vi "Display Thermocouple Data.vi"(0 "Sensor":T1={"Sensor Name"="AI 0", "Sensor Info"={"Manufacturer"="", "Model"="", "Serial Number"=""}, "Last Cal Info"={"Last Calibration Date"=3153138208.25, "Calibrator"="", "Cal Duration"=0}, "Voltage Range"={"High Limit"=0.0, "Low Limit"=10.0}, "EGU Range"={"High Limit"=0.0, "Low Limit"=10.0}, "Units"="Volts", "Calibration Type"=enum."Calibrate Analog", "EGU List"=[0.0, 10000.0], "Voltage List"=[0.0, 5.0], "Coefficients"=[3.658184866139891e-14, 1999.9999999999998], "Order"=1, "Algorithm"=enum."SVD", "Max Error % of Full Scale"=0.0, "Max Mean Squared Error"=0.0, "Use Error %"=FALSE, "Use MSE"=FALSE, "Allow Manual Entry"=FALSE, "Max Stability Error"=2.0, "Max Error % of Reading"=0.0, "Use Error % of Reading"=FALSE}, 1 "Shunt Cal":bool=TRUE, 5 "Channel Info":T2, 9 "Channel":string) -> (4 "Sensor out":T1)   [LabVIEW 2019]
uses:
  AI Read (waveform).vi
  AI Read (scaled array).vi
  <vilib>/Analysis/NI_AALBase.lvlib
  <vilib>/Analysis/baseanly.llb/Mean (DBL).vi
  <vilib>/Analysis/NI_AALPro.lvlib
  Type Defs and Controls/Channel Config Screen.ctl
panel:
  in  "Auto Shunt Cal Message":bool
  out "Temperature":dbl
  in  "OK":bool
  out "Sensor":string
  out "Channel Name":string
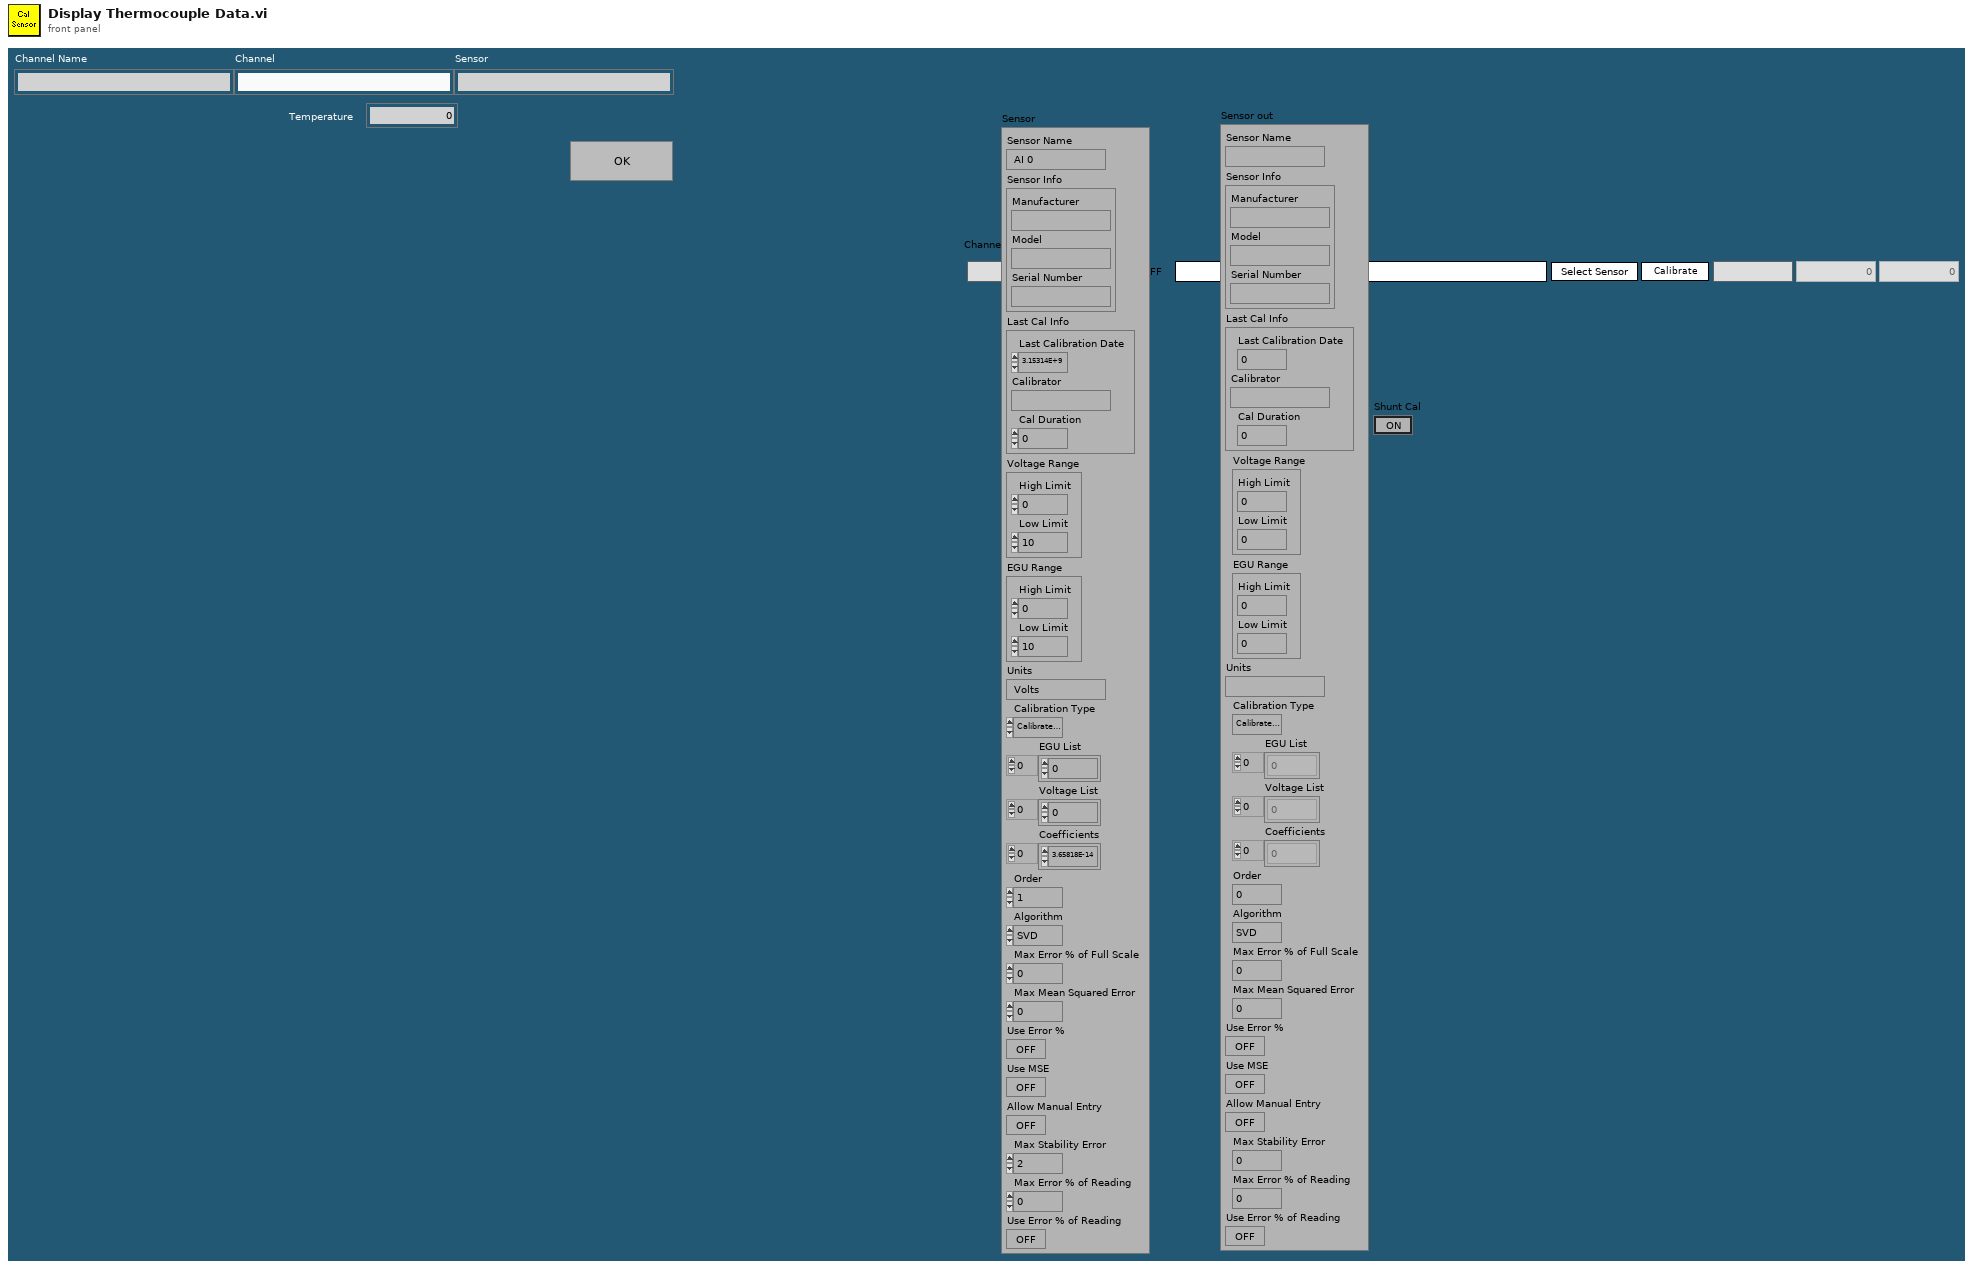
[diagram p1: front panel]
types:
  T1 = cluster{"Sensor Name":string, "Sensor Info":cluster{"Manufacturer":string, "Model":string, "Serial Number":string}, "Last Cal Info":cluster{"Last Calibration Date":dbl, "Calibrator":string, "Cal Duration":i32}, "Voltage Range":cluster{"High Limit":dbl, "Low Limit":dbl}, "EGU Range":cluster{"High Limit":dbl, "Low Limit":dbl}, "Units":string, "Calibration Type":enum16{"Calibrate Analog", "Compare Analog Calibration"}, "EGU List":dbl[], "Voltage List":dbl[], "Coefficients":dbl[], "Order":i32, "Algorithm":enum32{"SVD", "Givens", "Givens2", "Householder", "LU Decomposition", "Cholesky"}, "Max Error % of Full Scale":dbl, "Max Mean Squared Error":dbl, "Use Error %":bool, "Use MSE":bool, "Allow Manual Entry":bool, "Max Stability Error":dbl, "Max Error % of Reading":dbl, "Use Error % of Reading":bool}
  T2 = typedef "Channel Config Screen.ctl" = cluster{"Channel":string, "Description":string, "Acquire":bool, "Sensor":string, "Chg Sensor":bool, "Cal Date":string, "Offset":dbl, "Span":dbl, "Cal":bool, "Test Limits":bool, "Type":string, "Data Index":u32}
  T3 = cluster{"Channel Info":T2, "Channel":string, "Sensor":cluster{"Sensor Name":string, "Sensor Info":cluster{"Manufacturer":string, "Model":string, "Serial Number":string}, "Last Cal Info":cluster{"Last Calibration Date":dbl, "Calibrator":string, "Cal Duration":i32}, "Voltage Range":cluster{"High Limit":dbl, "Low Limit":dbl}, "EGU Range":cluster{"High Limit":dbl, "Low Limit":dbl}, "Units":string, "Calibration Type":enum16{"Calibrate Analog", "Compare Analog Calibration"}, "EGU List":dbl[], "Voltage List":dbl[], "Coefficients":dbl[], "Order":i32, "Algorithm":enum32{"SVD", "Givens", "Givens2", "Householder", "LU Decomposition", "Cholesky"}, "Max Error % of Full Scale":dbl, "Max Mean Squared Error":dbl, "Use Error %":bool, "Use MSE":bool, "Allow Manual Entry":bool, "Max Stability Error":dbl, "Max Error % of Reading":dbl, "Use Error % of Reading":bool}, "taskID":u32, "Allow Shunt Cal":bool}
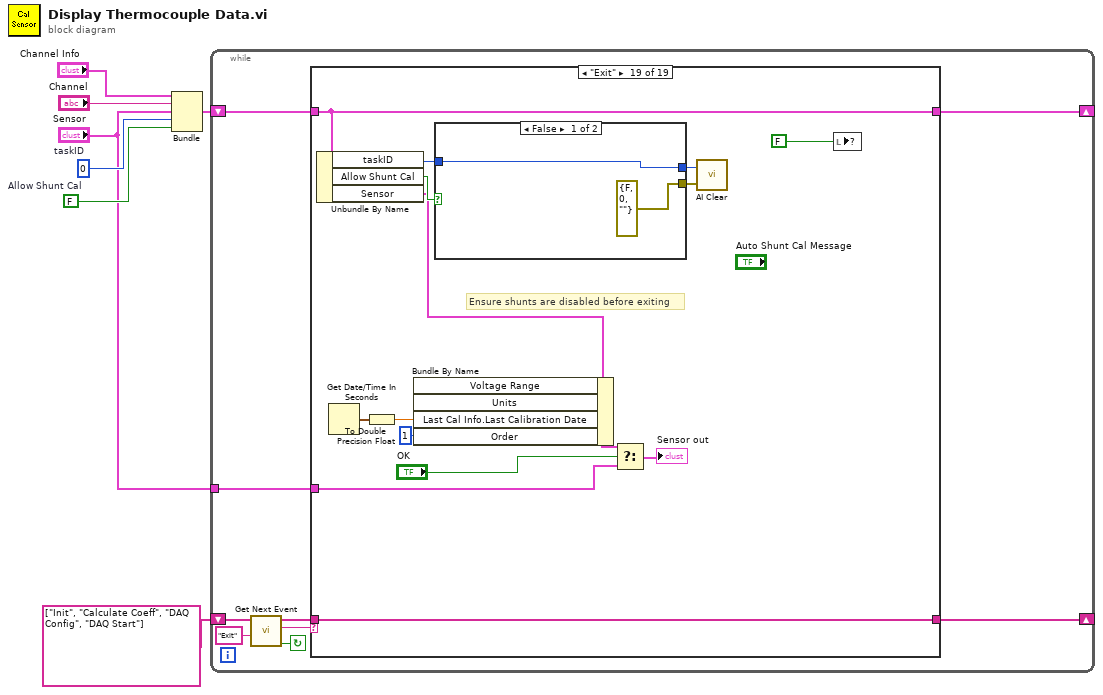
[diagram p0: block diagram]
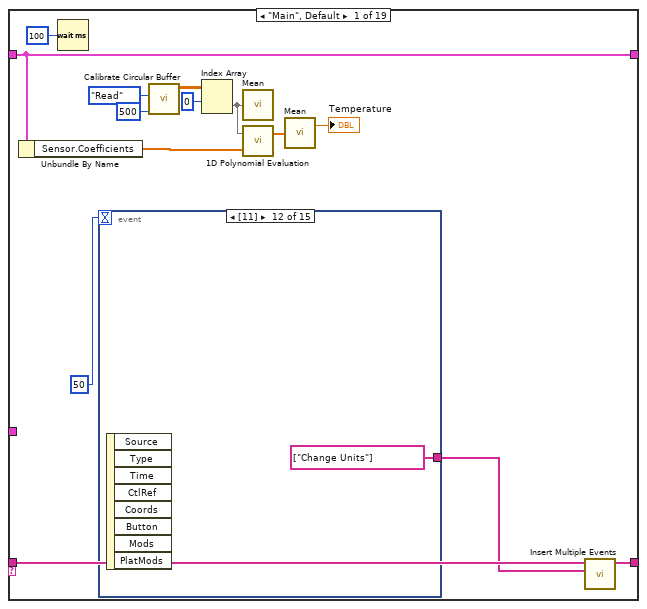
[diagram p2: hidden frame]
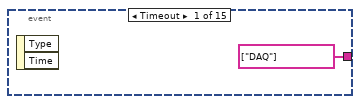
[diagram p3: hidden frame]
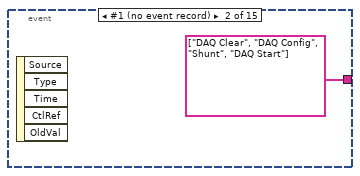
[diagram p4: hidden frame]
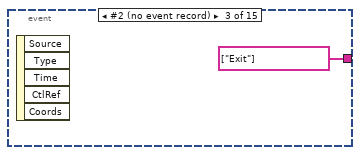
[diagram p5: hidden frame]
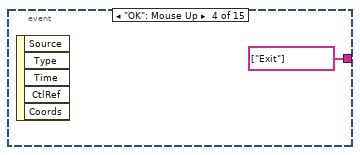
[diagram p6: hidden frame]
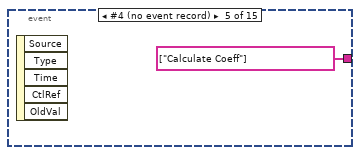
[diagram p7: hidden frame]
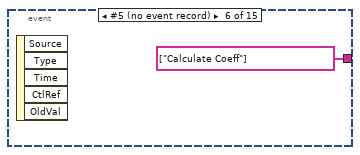
[diagram p8: hidden frame]
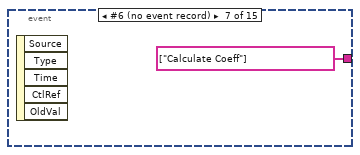
[diagram p9: hidden frame]
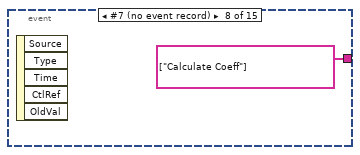
[diagram p10: hidden frame]
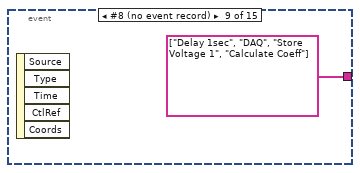
[diagram p11: hidden frame]
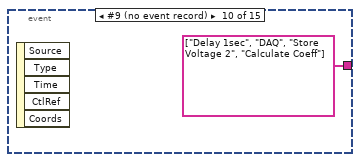
[diagram p12: hidden frame]
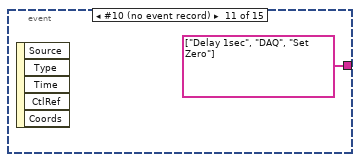
[diagram p13: hidden frame]
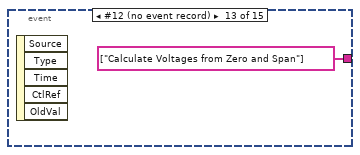
[diagram p14: hidden frame]
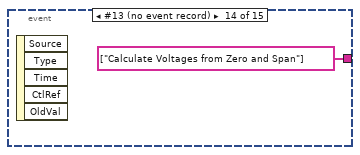
[diagram p15: hidden frame]
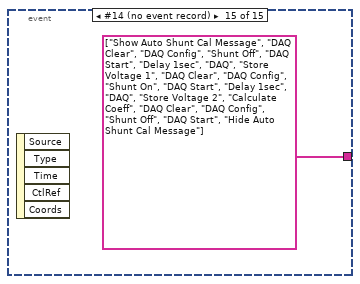
[diagram p16: hidden frame]
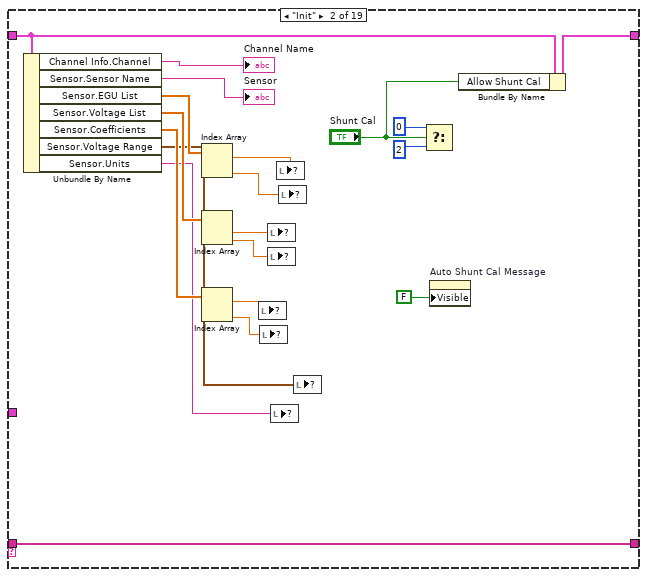
[diagram p17: hidden frame]
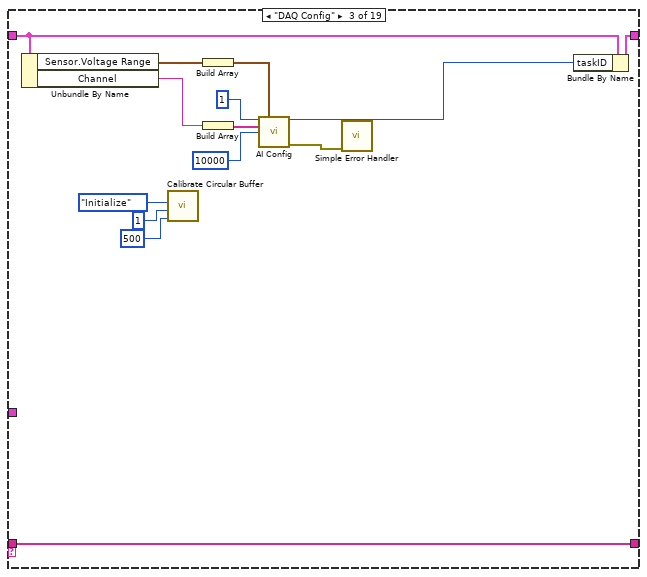
[diagram p18: hidden frame]
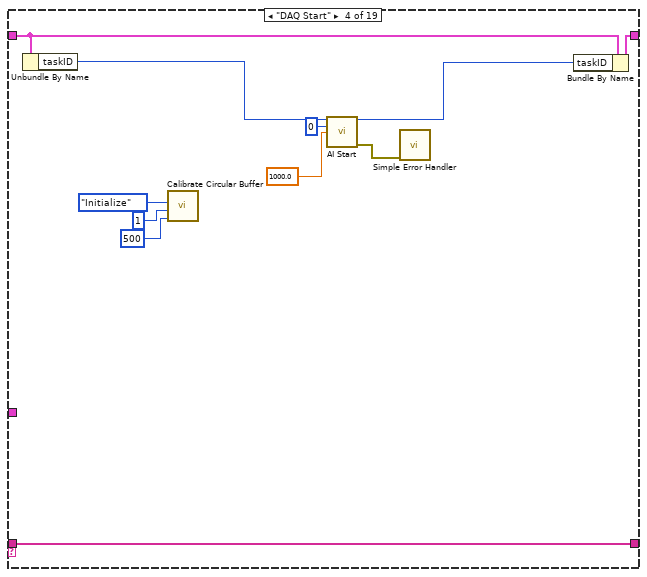
[diagram p19: hidden frame]
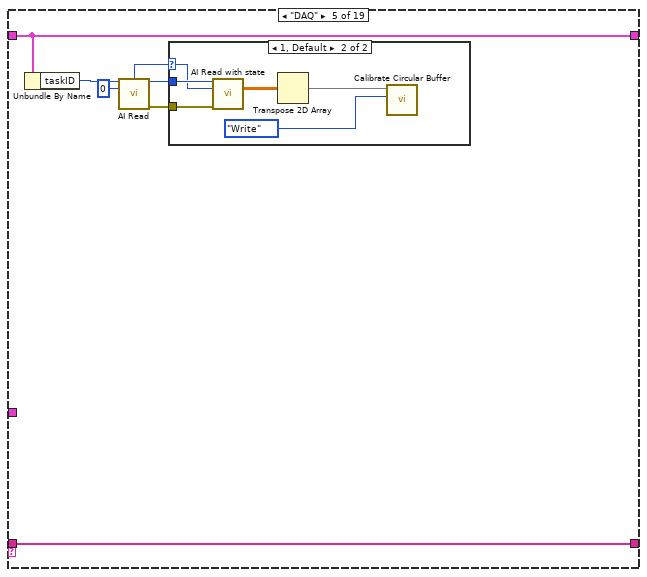
[diagram p20: hidden frame]
diagram:
  w3 = FALSE  # Allow Shunt Cal
  w5 = u32 0  # taskID
  n1 = Bundle("Channel Info"="Channel Info", "Channel"="Channel", "Sensor"="Sensor", "taskID"=w5, "Allow Shunt Cal"=w3) -> (w6:T3)  [unwired: 1 in]
  n2 = while {
    shift-left: string[] ["Init", "Calculate Coeff", "DAQ Config", "DAQ Start"] ("event queue out") -> [w14]
    shift-right: [w12] -> _
    shift-left: w6 -> [w13]
    shift-right: [w9] -> _
    tunnel: "Sensor" -> [w10]
    stop <- w16 continue-if-true
    n3 = call "Get Next Event.vi"("Exit Event"="Exit", "event queue in"=w14) -> ("Condition (Exit:F)"=w16:bool, "next event"=w15:string, "event queue out"=w8:string[])  [unwired: 3 in]
    n4 = case shown="\"Exit\"" w15 {
      tunnel: w13 -> [w21 w62 w76 w91 w99 w107 w115 w122 w129 w137 w144 w152 w160 w170 w175 w184 w194 w197 w213]
      tunnel: [w31 w65 w81 w92 w93 w108 w109 w117 w124 w141 w143 w151 w159 w163 w177 w186 w193 w196 w214] -> w12
      tunnel: w8 -> [w30 w65 w81 w92 w93 w108 w109 w117 w124 w141 w143 w151 w159 w162 w177 w186 w193 w196 w214]
      tunnel: w10 -> [_ _ _ _ _ _ _ _ _ _ _ _ _ _ _ _ _ _ w206]
      tunnel: [w21 w64 w75 w90 w99 w107 w115 w122 w129 w136 w144 w152 w160 w170 w176 w183 w194 w197 w213] -> w9
      frame "Main", Default {
        n5 = Unbundle By Name(w21) -> ("Sensor.Coefficients"=w17:dbl[])
        n6 = Wait (ms)(milliseconds to wait=u32 100) -> ()  [unwired: 1 out]
        n7 = event shown="[11]" {
          selector: _ -> [_ _ _ _ _ _ _ _ _ _ _ _ _ _ _]
          dyn-events: _ -> [_ _ _ _ _ _ _ _ _ _ _ _ _ _ _]
          timeout: 50 -> [_ _ _ _ _ _ _ _ _ _ _ _ _ _ _]
          tunnel: [string[] ["DAQ"] ("Events to Insert") string[] ["DAQ Clear", "DAQ Config", "Shunt", "DAQ Start"] ("Events to Insert") string[] ["Exit"] ("Events to Insert") string[] ["Exit"] ("Events to Insert") string[] ["Calculate Coeff"] ("Events to Insert") string[] ["Calculate Coeff"] ("Events to Insert") string[] ["Calculate Coeff"] ("Events to Insert") string[] ["Calculate Coeff"] ("Events to Insert") string[] ["Delay 1sec", "DAQ", "Store Voltage 1", "Calculate Coeff"] ("Events to Insert") string[] ["Delay 1sec", "DAQ", "Store Voltage 2", "Calculate Coeff"] ("Events to Insert") string[] ["Delay 1sec", "DAQ", "Set Zero"] ("Events to Insert") string[] ["Change Units"] ("Events to Insert") string[] ["Calculate Voltages from Zero and Span"] ("Events to Insert") string[] ["Calculate Voltages from Zero and Span"] ("Events to Insert") string[] ["Show Auto Shunt Cal Message", "DAQ Clear", "DAQ Config", "Shunt Off", "DAQ Start", "Delay 1sec", "DAQ", "Store Voltage 1", "DAQ Clear", "DAQ Config", "Shunt On", "DAQ Start", "Delay 1sec", "DAQ", "Store Voltage 2", "Calculate Coeff", "DAQ Clear", "DAQ Config", "Shunt Off", "DAQ Start", "Hide Auto Shunt Cal Message"] ("Events to Insert")] -> w28
          event Timeout {
            n8 = event-data() -> ()  [unwired: 1 in, 2 out]
          }
          event #1 (no event record) {
            n9 = event-data() -> ()  [unwired: 1 in, 5 out]
          }
          event #2 (no event record) {
            n10 = event-data() -> ()  [unwired: 1 in, 5 out]
          }
          event "OK": Mouse Up {
            n11 = event-data() -> ()  [unwired: 1 in, 5 out]
          }
          event #4 (no event record) {
            n12 = event-data() -> ()  [unwired: 1 in, 5 out]
          }
          event #5 (no event record) {
            n13 = event-data() -> ()  [unwired: 1 in, 5 out]
          }
          event #6 (no event record) {
            n14 = event-data() -> ()  [unwired: 1 in, 5 out]
          }
          event #7 (no event record) {
            n15 = event-data() -> ()  [unwired: 1 in, 5 out]
          }
          event #8 (no event record) {
            n16 = event-data() -> ()  [unwired: 1 in, 5 out]
          }
          event #9 (no event record) {
            n17 = event-data() -> ()  [unwired: 1 in, 5 out]
          }
          event #10 (no event record) {
            n18 = event-data() -> ()  [unwired: 1 in, 5 out]
          }
          event #11 (no event record) {
            n19 = event-data() -> ()  [unwired: 1 in, 8 out]
          }
          event #12 (no event record) {
            n20 = event-data() -> ()  [unwired: 1 in, 5 out]
          }
          event #13 (no event record) {
            n21 = event-data() -> ()  [unwired: 1 in, 5 out]
          }
          event #14 (no event record) {
            n22 = event-data() -> ()  [unwired: 1 in, 5 out]
          }
        }
        n23 = call "Calibrate Circular Buffer.vi"("# of Samples"=500, "Mode"=enum16{"Initialize", "Read", "Write"}."Read") -> ("Data Read"=w25:sgl[][])  [unwired: 7 in, 2 out]
        n24 = Index Array(array=w25, index (row)=0) -> (element=w20:sgl[])  [unwired: 1 in]
        n25 = call-poly <vilib>:"Mean.vi"("X"=w20) -> ("mean"=w23:dbl)  [unwired: 1 out]
        n26 = call <vilib>:"1D Polynomial Evaluation.vi"("Coefficients: a"=w17, "X"=w20) -> ("Y"=w19:dbl[])  [unwired: 1 out]
        n27 = call-poly <vilib>:"Mean.vi"("X"=w19) -> ("mean"=→"Temperature":dbl)  [unwired: 1 out]
        n28 = call "Insert Multiple Events.vi"("Events to Insert"=w28, "Event queue in"=w30) -> ("Event queue out"=w31:string[])  [unwired: 5 in]
      }
      frame "Init" {
        n29 = Unbundle By Name(w62) -> ("Channel Info.Channel"=→"Channel Name":string, "Sensor.Sensor Name"=→"Sensor":string, "Sensor.EGU List"=w59:dbl[], "Sensor.Voltage List"=w56:dbl[], "Sensor.Coefficients"=w51:dbl[], "Sensor.Voltage Range"=w48:cluster{"High Limit":dbl, "Low Limit":dbl}, "Sensor.Units"=w47:string)
        n30 = Index Array(array=w59) -> (element #1=w58:dbl, element #2=w57:dbl)  [unwired: 2 in]
        n31 = Index Array(array=w56) -> (element #1=w55:dbl, element #2=w54:dbl)  [unwired: 2 in]
        n32 = Index Array(array=w51) -> (element #1=w53:dbl, element #2=w52:dbl)  [unwired: 2 in]
        n33 = local write item#-1(w53) -> ()
        n34 = local write item#-1(w52) -> ()
        n35 = local write item#-1(w55) -> ()
        n36 = local write item#-1(w54) -> ()
        n37 = local write item#-1(w47) -> ()
        n38 = local write item#-1(w58) -> ()
        n39 = local write item#-1(w57) -> ()
        n40 = local write item#-1(w48) -> ()
        n41 = Select(t=u8 0 ("Disabled"), s="Shunt Cal", f=u8 2 ("Disabled")) -> (s? t:f=w50:u8)
        n42 = property on="Auto Shunt Cal Message" class="Bool"("Visible"=FALSE) -> ()  [unwired: 2 in, 2 out]
        n43 = Bundle By Name(cluster=w62, "Allow Shunt Cal"="Shunt Cal") -> (w64:T3)
      }
      frame "DAQ Config" {
        n44 = Unbundle By Name(w76) -> ("Sensor.Voltage Range"=w78:cluster{"High Limit":dbl, "Low Limit":dbl}, "Channel"=w73:string)
        n45 = call "Calibrate Circular Buffer.vi"("# of Samples"=500, "# of Channels"=1, "Mode"=enum16{"Initialize", "Read", "Write"}."Initialize") -> ()  [unwired: 6 in, 3 out]
        n46 = Build Array(w78) -> (w77:cluster{"High Limit":dbl, "Low Limit":dbl}[])
        n47 = Build Array(w73) -> (w74:string[])
        n48 = call "AI Config.vi"("device (1)"=i16 1, "input limits (no change)"=w77, "channels (0)"=w74, "buffer size (1000 scans)"=10000) -> ("taskID"=w69:u32, "error out"=w68:errorcluster)  [unwired: 9 in, 1 out]
        n49 = call <vilib>:"Simple Error Handler.vi"("error in (no error)"=w68) -> ()  [unwired: 4 in, 5 out]
        n50 = Bundle By Name(cluster=w76, "taskID"=w69) -> (w75:T3)
      }
      frame "DAQ Start" {
        n51 = Unbundle By Name(w91) -> ("taskID"=w83:u32)
        n52 = call "Calibrate Circular Buffer.vi"("# of Samples"=500, "# of Channels"=1, "Mode"=enum16{"Initialize", "Read", "Write"}."Initialize") -> ()  [unwired: 6 in, 3 out]
        n53 = call "AI Start.vi"("taskID in"=w83, "number of scans to acquire (-1)"=0, "scan rate (1000 scans/sec)"=sgl 1000.0) -> ("taskID out"=w85:u32, "error out"=w82:errorcluster)  [unwired: 9 in, 2 out]
        n54 = call <vilib>:"Simple Error Handler.vi"("error in (no error)"=w82) -> ()  [unwired: 4 in, 5 out]
        n55 = Bundle By Name(cluster=w91, "taskID"=w85) -> (w90:T3)
      }
      frame "DAQ" {
        n56 = Unbundle By Name(w99) -> ("taskID"=w98:u32)
        n57 = call-poly "AI Read.vi"("taskID in"=w98, "number of scans to read (-1:all)"=0) -> ("scan backlog"=w96:u32, "taskID out"=w95:u32, "error out"=w94:errorcluster)  [unwired: 8 in, 3 out]
        n58 = case shown="1, Default" w96 {
          selector: w96 -> [_ w103]
          tunnel: w95 -> [_ w105]
          tunnel: w94 -> [_ w104]
          frame 0 {
          }
          frame 1, Default {
            n59 = call-poly "AI Read with state .vi"("taskID in"=w105, "number of scans to read (-1:all)"=w103, "error in (no error)"=w104) -> ("scaled data"=w102:sgl[][])  [unwired: 7 in, 5 out]
            n60 = Transpose 2D Array(2D array=w102) -> (transposed array=w100:sgl[][])
            n61 = call "Calibrate Circular Buffer.vi"("Mode"=enum16{"Initialize", "Read", "Write"}."Write", "Data to Write"=w100) -> ()  [unwired: 7 in, 3 out]
          }
        }
      }
      frame "DAQ Clear" {
        n62 = Unbundle By Name(w107) -> ("taskID"=w106:u32)
        n63 = call "AI Clear.vi"("taskID in"=w106) -> ()  [unwired: 5 in, 2 out]
      }
      frame "Shunt" {
        w113 = u16 25 items=["Notch Filter Frequency", "Measurement Mode", "Open Thermocouple detection", "Ground Referencing", "Probe Attenuation", "Actual RIS Count", "Total Number of Physical Total Time Bins", "Minimal RIS Count", "Maximal Oversampling", "Maximal Scan Rate", "Scope Acquisition Type", "Conversions per Measurement", "Autozero", "SCXI Gain", "Filter Setting", "SCXI External Filter Clock", "SCXI OutClk Divider", "SCXI DC Voltage Excitation", "SCXI DC Current Excitation", "SCXI Connection Type", "SCXI AC Voltage Excitation", "SCXI AC Frequency Excitation", "SCXI Synchronization Type", "SCXI Fine Potentiometer", "SCXI Course Potentiometer", "SCXI Shunt A Enabled", "SCXI Shunt B Enabled", "Measurement Setup Time", "Measurement Total Time", "DSA On-board Excitation", "FIFO Transfer Count"] ("parameter name")
        w112 = u16 0 items=["Set", "Get", "Translate"] ("operation")
        n64 = Unbundle By Name(w115) -> ("taskID"=w114:u32)  [unwired: 1 out]
        n65 = call "AI Parameter.vi"("task ID in"=w114, "operation"=w112, "parameter name"=w113) -> ("boolean in"=w111:bool, "error out"=w110:errorcluster)  [unwired: 10 in, 5 out]
        n66 = call <vilib>:"Simple Error Handler.vi"("error in (no error)"=w110) -> ()  [unwired: 4 in, 5 out]
      }
      frame "Shunt On" {
        w120 = u16 25 items=["Notch Filter Frequency", "Measurement Mode", "Open Thermocouple detection", "Ground Referencing", "Probe Attenuation", "Actual RIS Count", "Total Number of Physical Total Time Bins", "Minimal RIS Count", "Maximal Oversampling", "Maximal Scan Rate", "Scope Acquisition Type", "Conversions per Measurement", "Autozero", "SCXI Gain", "Filter Setting", "SCXI External Filter Clock", "SCXI OutClk Divider", "SCXI DC Voltage Excitation", "SCXI DC Current Excitation", "SCXI Connection Type", "SCXI AC Voltage Excitation", "SCXI AC Frequency Excitation", "SCXI Synchronization Type", "SCXI Fine Potentiometer", "SCXI Course Potentiometer", "SCXI Shunt A Enabled", "SCXI Shunt B Enabled", "Measurement Setup Time", "Measurement Total Time", "DSA On-board Excitation", "FIFO Transfer Count"] ("parameter name")
        w119 = u16 0 items=["Set", "Get", "Translate"] ("operation")
        n67 = Unbundle By Name(w122) -> ("taskID"=w121:u32)  [unwired: 1 out]
        n68 = call "AI Parameter.vi"("task ID in"=w121, "operation"=w119, "parameter name"=w120, "boolean in"=TRUE) -> ("error out"=w118:errorcluster)  [unwired: 10 in, 5 out]
        n69 = call <vilib>:"Simple Error Handler.vi"("error in (no error)"=w118) -> ()  [unwired: 4 in, 5 out]
      }
      frame "Shunt Off" {
        w127 = u16 25 items=["Notch Filter Frequency", "Measurement Mode", "Open Thermocouple detection", "Ground Referencing", "Probe Attenuation", "Actual RIS Count", "Total Number of Physical Total Time Bins", "Minimal RIS Count", "Maximal Oversampling", "Maximal Scan Rate", "Scope Acquisition Type", "Conversions per Measurement", "Autozero", "SCXI Gain", "Filter Setting", "SCXI External Filter Clock", "SCXI OutClk Divider", "SCXI DC Voltage Excitation", "SCXI DC Current Excitation", "SCXI Connection Type", "SCXI AC Voltage Excitation", "SCXI AC Frequency Excitation", "SCXI Synchronization Type", "SCXI Fine Potentiometer", "SCXI Course Potentiometer", "SCXI Shunt A Enabled", "SCXI Shunt B Enabled", "Measurement Setup Time", "Measurement Total Time", "DSA On-board Excitation", "FIFO Transfer Count"] ("parameter name")
        w126 = u16 0 items=["Set", "Get", "Translate"] ("operation")
        n70 = Unbundle By Name(w129) -> ("taskID"=w128:u32)  [unwired: 1 out]
        n71 = call "AI Parameter.vi"("task ID in"=w128, "operation"=w126, "parameter name"=w127, "boolean in"=FALSE) -> ("error out"=w125:errorcluster)  [unwired: 10 in, 5 out]
        n72 = call <vilib>:"Simple Error Handler.vi"("error in (no error)"=w125) -> ()  [unwired: 4 in, 5 out]
      }
      frame "Calculate Coeff" {
        n73 = Build Array() -> (w134:void[], w140:dbl)  [unwired: 1 in]
        n74 = Build Array() -> (w133:void[], w138:dbl, w139:dbl)
        n75 = call <vilib>:"Linear Fit Coefficients.vi"("Y"=w134, "X"=w133) -> ("slope"=w132:dbl, "intercept"=w131:dbl)  [unwired: 11 in, 1 out]
        n76 = Build Array(w131, w132) -> (w135:dbl[])
        n77 = local write item#-1(w131) -> ()
        n78 = local write item#-1(w132) -> ()
        n79 = Bundle By Name(cluster=w137, "Sensor.EGU List"=w134, "Sensor.Voltage List"=w133, "Sensor.Coefficients"=w135, "Sensor.Order"=1) -> (w136:T3)
      }
      frame "Delay 1sec" {
        n80 = Wait (ms)(milliseconds to wait=u32 1000) -> ()  [unwired: 1 out]
      }
      frame "Store Voltage 1" {
        n81 = call "Calibrate Circular Buffer.vi"("# of Samples"=500, "Mode"=enum16{"Initialize", "Read", "Write"}."Read") -> ("Data Read"=w148:sgl[][])  [unwired: 7 in, 2 out]
        n82 = Index Array(array=w148, index (row)=0) -> (element=w146:sgl[])  [unwired: 1 in]
        n83 = call-poly <vilib>:"Mean.vi"("X"=w146) -> ("mean"=w145:dbl)  [unwired: 1 out]
        n84 = local write item#-1(w145) -> ()
      }
      frame "Store Voltage 2" {
        n85 = call "Calibrate Circular Buffer.vi"("# of Samples"=500, "Mode"=enum16{"Initialize", "Read", "Write"}."Read") -> ("Data Read"=w156:sgl[][])  [unwired: 7 in, 2 out]
        n86 = Index Array(array=w156, index (row)=0) -> (element=w154:sgl[])  [unwired: 1 in]
        n87 = call-poly <vilib>:"Mean.vi"("X"=w154) -> ("mean"=w153:dbl)  [unwired: 1 out]
        n88 = local write item#-1(w153) -> ()
      }
      frame "Set Zero" {
        n89 = call "Calibrate Circular Buffer.vi"("# of Samples"=500, "Mode"=enum16{"Initialize", "Read", "Write"}."Read") -> ("Data Read"=w167:sgl[][])  [unwired: 7 in, 2 out]
        n90 = Index Array(array=w167, index (row)=0) -> (element=w165:sgl[])  [unwired: 1 in]
        n91 = call-poly <vilib>:"Mean.vi"("X"=w165) -> ("mean"=w164:dbl)  [unwired: 1 out]
        n92 = local write item#-1(w164) -> ()
        n93 = call "Insert Multiple Events.vi"("Events to Insert"=string[] ["Calculate Voltages from Zero and Span"], "Event queue in"=w162) -> ("Event queue out"=w163:string[])  [unwired: 5 in]
      }
      frame "Change Units" {
        n94 = Unbundle By Name(w175) -> ("Sensor.Units"=w174:string)
        n95 = call "Select Units.vi"() -> ("Element"=w172:string, "Cancelled"=w173:bool)  [unwired: 4 in]
        n96 = Select(t=w174, s=w173, f=w172) -> (s? t:f=w171:string)
        n97 = local write item#-1(w171) -> ()
        n98 = Bundle By Name(cluster=w175, "Sensor.Units"=w171) -> (w176:T3)
      }
      frame "Calculate Voltages from Zero and Span" {
        n99 = Unbundle By Name(w184) -> ("Sensor.EGU List"=w185:dbl[])
        n100 = for {
          tunnel: w185 -> [w191] mode=indexing
          tunnel: [w189] -> w182 mode=indexing
          tunnel: [w190] -> w179
          tunnel: [w187] -> w178
          n101 = Subtract(x=w191, y=w190) -> (x-y=w188:dbl)
          n102 = Divide(x=w188, y=w187) -> (x/y=w189:dbl)
        }
        n103 = Index Array(array=w182) -> (element #1=w181:dbl, element #2=w180:dbl)  [unwired: 2 in]
        n104 = Bundle By Name(cluster=w184, "Sensor.Voltage List"=w182) -> (w183:T3)
        n105 = local write item#-1(w181) -> ()
        n106 = local write item#-1(w180) -> ()
      }
      frame "Show Auto Shunt Cal Message" {
        n107 = property on="Auto Shunt Cal Message" class="Bool"("Visible"=TRUE) -> ()  [unwired: 2 in, 2 out]
      }
      frame "Hide Auto Shunt Cal Message" {
        n108 = property on="Auto Shunt Cal Message" class="Bool"("Visible"=FALSE) -> ()  [unwired: 2 in, 2 out]
      }
      frame "Exit" {
        # "Ensure shunts are disabled before exiting"
        n109 = Unbundle By Name(w213) -> ("taskID"=w212:u32, "Allow Shunt Cal"=w209:bool, "Sensor"=w204:T1)
        n110 = Get Date/Time In Seconds() -> (seconds since 1Jan1904=w202:timestamp)
        n111 = To Double Precision Float(number=w202) -> (double precision float=w201:dbl)
        n112 = Bundle By Name(cluster=w204, "Last Cal Info.Last Calibration Date"=w201, "Order"=1) -> (w203:T1, "Voltage Range"=w198:cluster{"High Limit":dbl, "Low Limit":dbl}, "Units"=w199:string)
        n113 = case shown="False" w209 {
          tunnel: w212 -> [w216 w220]
          tunnel: [w216 w218] -> w211
          tunnel: [errorcluster {"status"=FALSE, "code"=0, "source"=""} ("error out") w217] -> w210
          frame False {
          }
          frame True {
            w221 = u16 25 items=["Notch Filter Frequency", "Measurement Mode", "Open Thermocouple detection", "Ground Referencing", "Probe Attenuation", "Actual RIS Count", "Total Number of Physical Total Time Bins", "Minimal RIS Count", "Maximal Oversampling", "Maximal Scan Rate", "Scope Acquisition Type", "Conversions per Measurement", "Autozero", "SCXI Gain", "Filter Setting", "SCXI External Filter Clock", "SCXI OutClk Divider", "SCXI DC Voltage Excitation", "SCXI DC Current Excitation", "SCXI Connection Type", "SCXI AC Voltage Excitation", "SCXI AC Frequency Excitation", "SCXI Synchronization Type", "SCXI Fine Potentiometer", "SCXI Course Potentiometer", "SCXI Shunt A Enabled", "SCXI Shunt B Enabled", "Measurement Setup Time", "Measurement Total Time", "DSA On-board Excitation", "FIFO Transfer Count"] ("parameter name")
            w222 = u16 0 items=["Set", "Get", "Translate"] ("operation")
            n114 = call "AI Parameter.vi"("task ID in"=w220, "operation"=w222, "parameter name"=w221, "boolean in"=TRUE) -> ("task ID out"=w218:u32, "error out"=w217:errorcluster)  [unwired: 10 in, 4 out]
          }
        }
        n115 = Select(t=w203, s="OK", f=w206) -> (s? t:f=→"Sensor out":T1)
        n116 = call "AI Clear.vi"("error in (no error)"=w210, "taskID in"=w211) -> ()  [unwired: 4 in, 2 out]
        n117 = local write item#-1(FALSE ("Auto Shunt Cal")) -> ()
      }
    }
  }
